vi "udp_init.vi"(8 "error in":errorcluster, 9 "Port In":u16, 10 "Local Timeout (ms)":i32) -> (0 "error out":errorcluster, 1 "Port Out":u16, 2 "connection ID":refnum<k16>)   [LabVIEW 2014]
panel:
  # "UDP Initialize"
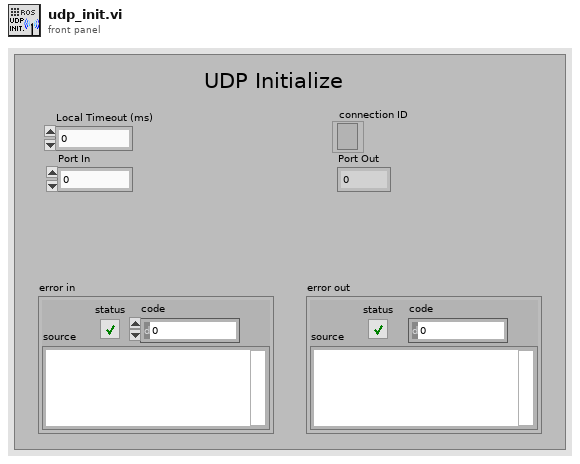
[diagram p1: front panel]
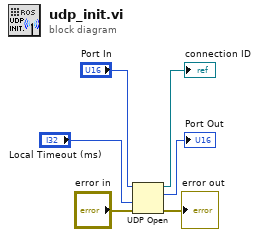
[diagram p0: block diagram]
diagram:
  n1 = UDP Open(8:"error in", 9:"Local Timeout (ms)", 11:"Port In") -> (port=→"connection ID":refnum<k16>, 0:→"error out":errorcluster, 2:→"Port Out":u16)  [unwired: 2 in]
